vi "Main.vi"(8 "error in":errorcluster, 11 "Acquire in":refnum<class "DataAcquire Worker.lvclass">) -> (0 "error out":errorcluster, 3 "Acquire out":refnum<class "DataAcquire Worker.lvclass">)   [LabVIEW 2018, in "DataAcquire Worker.lvclass"]
doc: "The Queued Message Handler of a Worker."
uses:
  DataAcquire Worker.lvclass
  D:/Program Files (x86)/National Instruments/LabVIEW 2018/vi.lib/addons/_Workers/Library/Classes/Worker/Worker.lvclass
  DataAcquire Worker.lvclass/DataAcquire Worker.ctl
  Initialization Data.ctl
  <vilib>/addons/_Workers/Library/Classes/Message Queue/Message Queue.lvclass
  <vilib>/addons/_Workers/Library/Classes/Worker/Worker.lvclass/Worker.ctl
  DataSave Worker/DataSave Worker.lvclass
  <vilib>/addons/_Workers/Library/Classes/Message/Enqueue Message to Self v2.vi
  <vilib>/addons/_Workers/Library/Classes/Message/Enqueue Message to Queue.vi
  <vilib>/addons/_Workers/Library/Classes/Message/Message.lvclass
  ChartView Worker/ChartView Worker.lvclass
  D:/Program Files (x86)/National Instruments/LabVIEW 2018/vi.lib/addons/_Workers/Library/Classes/Workers Object/Workers Object.lvclass
  <vilib>/addons/_Workers/Library/Classes/Worker/Worker.lvclass
types:
  T1 = typedef "DataAcquire Worker.lvclass/Initialization Data.ctl" = cluster{"String":string, "Chart Queue":refnum<class "Message Queue.lvclass">}
  T2 = typedef "Workers.lvlib/Case Label.ctl" = string
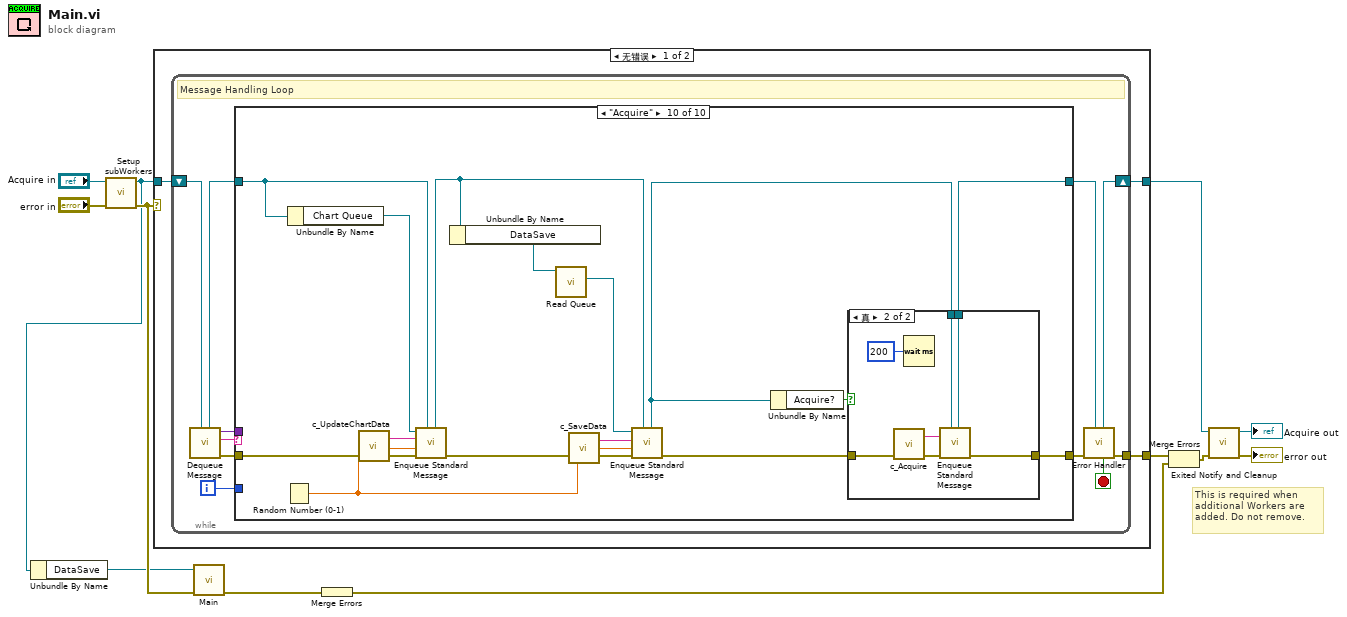
[diagram p0: block diagram]
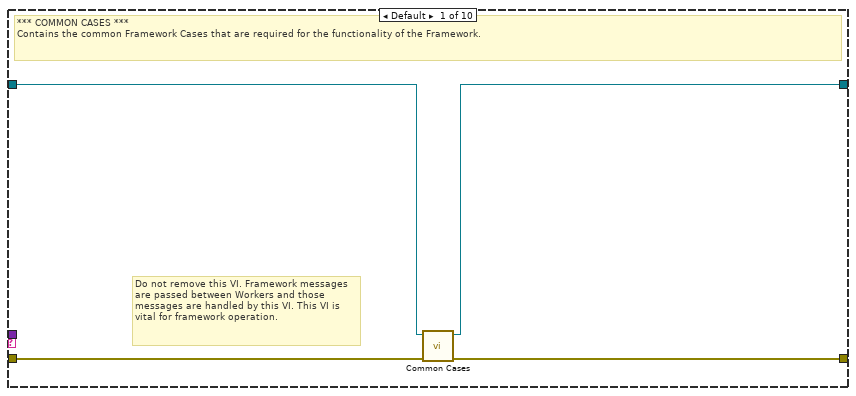
[diagram p2: hidden frame]
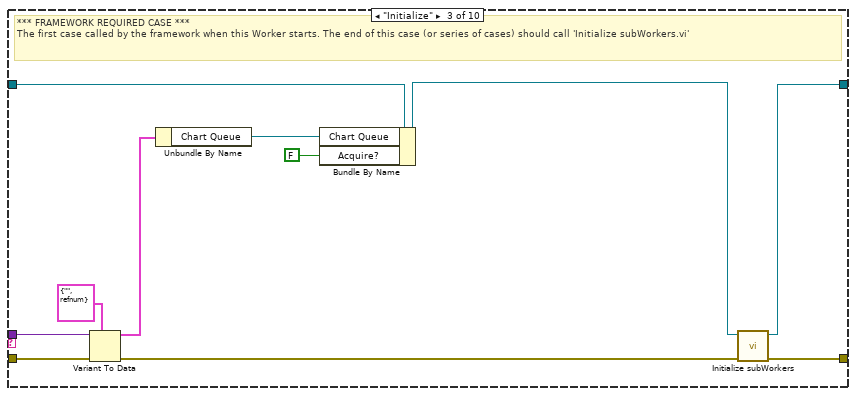
[diagram p4: hidden frame]
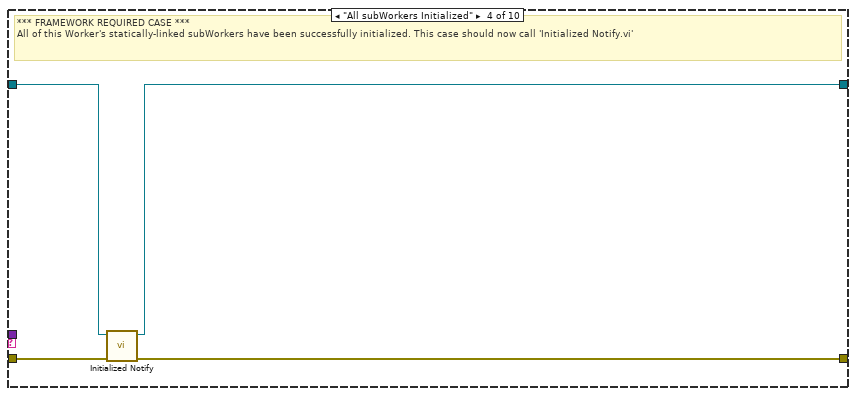
[diagram p5: hidden frame]
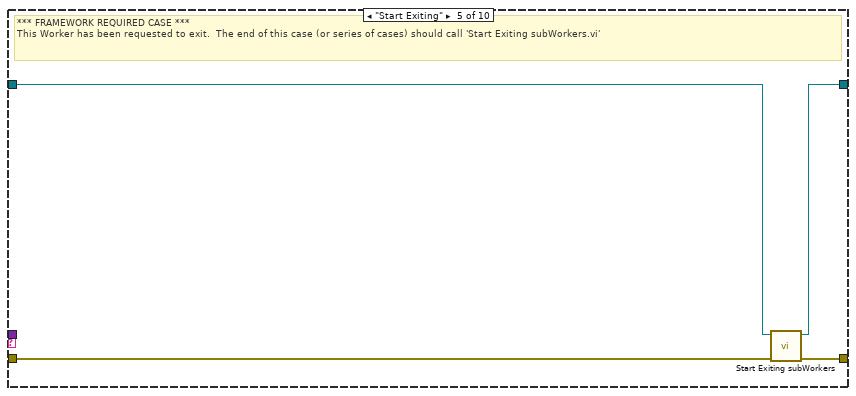
[diagram p6: hidden frame]
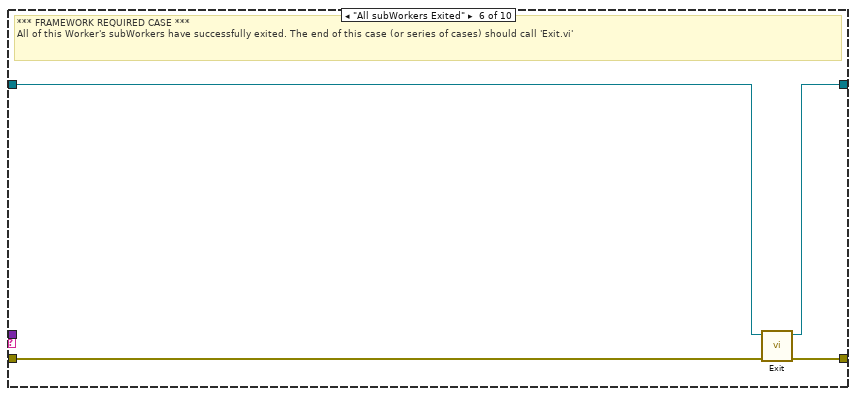
[diagram p7: hidden frame]
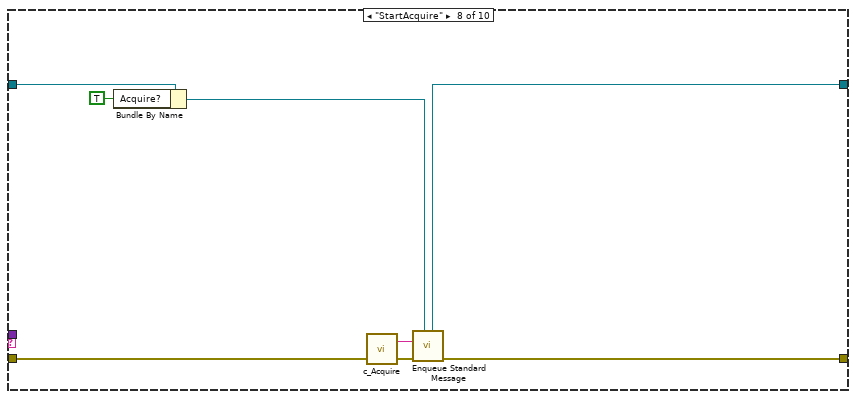
[diagram p9: hidden frame]
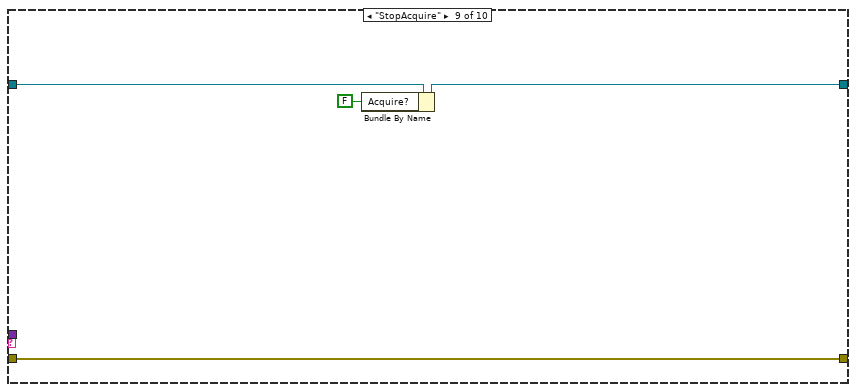
[diagram p10: hidden frame]
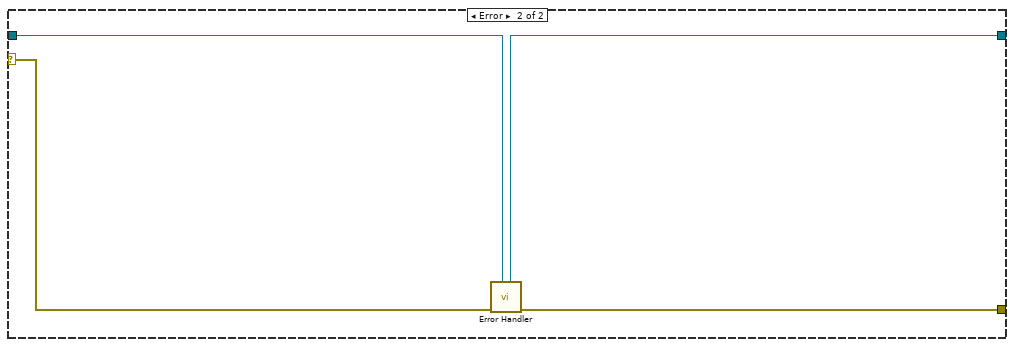
[diagram p12: hidden frame]
diagram:
  # "This is required when additional Workers are added. Do not remove."
  n1 = call "Setup subWorkers.vi"("error in"="error in", "DataAcquire Worker in"="Acquire in") -> ("error out"=w6:errorcluster, "DataAcquire Worker out"=w4:refnum<class "DataAcquire Worker.lvclass">)  [unwired: 8 in]
  n2 = Unbundle By Name(w4) -> ("DataSave"=w1:refnum<class "DataSave Worker.lvclass">)
  n3 = case shown="无错误" w6 {
    tunnel: w4 -> [w13 w93]
    tunnel: [w15 w94] -> w11
    tunnel: [w14 w92] -> w12
    selector: w6 -> [_ w95]
    frame No Error {
      n4 = while {
        shift-right: [w24] -> w14
        shift-left: w13 -> [w26]
        tunnel: [w25] -> w15
        i -> [w16]
        stop <- w17 stop-if-true
        # "Message Handling Loop"
        n5 = call-dynamic "Dequeue Message.vi"("Worker"=w26) -> ("error out"=w23:errorcluster, "Case out"=w18:string, "Data out"=w19:variant, "Worker out"=w21:refnum<class "DataAcquire Worker.lvclass">)  [unwired: 6 in, 1 out]
        n6 = case "Worker MHL Case Structure (DO NOT CHANGE LABEL NAME)" shown="\"Acquire\"" w18 {
          tunnel: w23 -> [w30 w31 w41 w47 w48 w55 w56 w64 w68 w78]
          tunnel: [w29 w31 w43 w45 w51 w54 w56 w61 w68 w83] -> w22
          tunnel: w21 -> [w28 w32 w40 w46 w49 w53 w57 w63 w67 w80]
          tunnel: [w27 w32 w42 w44 w50 w52 w57 w59 w66 w82] -> w20
          tunnel: w19 -> [_ _ w39 _ _ _ _ _ _ _]
          tunnel: w16 -> [_ _ _ _ _ _ _ _ _ _]
          frame Default {
            # "Do not remove this VI. Framework messages are passed between Workers and those messages are handled by this VI. This VI is vital for framework operation."
            # "*** COMMON CASES ***\nContains the common Framework Cases that are required for the functionality of the Framework."
            n7 = call-dynamic "Common Cases.vi"("error in"=w30, "Worker in"=w28) -> ("error out"=w29:errorcluster, "Worker out"=w27:refnum<class "DataAcquire Worker.lvclass">)  [unwired: 8 in]
          }
          frame "------ FRAMEWORK REQUIRED CASES ------" {
            # "Start of Framework Required Cases"
          }
          frame "Initialize" {
            # "*** FRAMEWORK REQUIRED CASE ***\nThe first case called by the framework when this Worker starts. The end of this case (or series of cases) should call 'Initialize subWorkers.vi'"
            n8 = Variant To Data(error in=w41, type=T1 {"String"="", "Chart Queue"=refnum} ("Cluster"), Variant=w39) -> (data=w36:T1, error out=w35:errorcluster)
            n9 = Unbundle By Name(w36) -> ("Chart Queue"=w34:refnum<class "Message Queue.lvclass">)
            n10 = Bundle By Name ("按名称捆绑")(cluster=w40, "Chart Queue"=w34, "Acquire?"=FALSE) -> (w37:refnum<class "DataAcquire Worker.lvclass">)
            n11 = call-dynamic "Initialize subWorkers.vi"("error in"=w35, "Worker"=w37) -> ("error out"=w43:errorcluster, "dup Worker out"=w42:refnum<class "DataAcquire Worker.lvclass">)  [unwired: 8 in]
          }
          frame "All subWorkers Initialized" {
            # "*** FRAMEWORK REQUIRED CASE ***\nAll of this Worker's statically-linked subWorkers have been successfully initialized. This case should now call 'Initialized Notify.vi'"
            n12 = call-dynamic "Initialized Notify.vi"("error in"=w47, "Worker"=w46) -> ("error out"=w45:errorcluster, "dup Worker out"=w44:refnum<class "DataAcquire Worker.lvclass">)  [unwired: 8 in]
          }
          frame "Start Exiting" {
            # "*** FRAMEWORK REQUIRED CASE ***\nThis Worker has been requested to exit.  The end of this case (or series of cases) should call 'Start Exiting subWorkers.vi'"
            n13 = call-dynamic "Start Exiting subWorkers.vi"("error_in"=w48, "Worker"=w49) -> ("error out"=w51:errorcluster, "dup Worker out"=w50:refnum<class "DataAcquire Worker.lvclass">)  [unwired: 8 in]
          }
          frame "All subWorkers Exited" {
            # "*** FRAMEWORK REQUIRED CASE ***\nAll of this Worker's subWorkers have successfully exited. The end of this case (or series of cases) should call 'Exit.vi'"
            n14 = call-dynamic "Exit.vi"("error_in"=w55, "Worker"=w53) -> ("error out"=w54:errorcluster, "dup Worker out"=w52:refnum<class "DataAcquire Worker.lvclass">)  [unwired: 8 in]
          }
          frame "-----------------------------------------------" {
            # "End of Framework Required Cases"
          }
          frame "StartAcquire" {
            n15 = Bundle By Name ("按名称捆绑")(cluster=w63, "Acquire?"=TRUE) -> (w60:refnum<class "DataAcquire Worker.lvclass">)
            n16 = call "c_Acquire.vi"() -> ("Case Label"=w58:T2)  [unwired: 1 in]
            n17 = call-poly <vilib>:"Enqueue Standard Message.vi"("Worker"=w60, "error in"=w64, "Case Label"=w58) -> ("error out"=w61:errorcluster, "dup Worker out"=w59:refnum<class "DataAcquire Worker.lvclass">)  [unwired: 7 in]
          }
          frame "StopAcquire" {
            n18 = Bundle By Name ("按名称捆绑")(cluster=w67, "Acquire?"=FALSE) -> (w66:refnum<class "DataAcquire Worker.lvclass">)
          }
          frame "Acquire" {
            n19 = Random Number (0-1)() -> (number: 0 to 1=w70:dbl)
            n20 = Unbundle By Name(w80) -> ("Chart Queue"=w79:refnum<class "Message Queue.lvclass">)
            n21 = call "c_UpdateChartData.vi"() -> ("Case Label"=w76:T2)  [unwired: 1 in]
            n22 = call-poly <vilib>:"Enqueue Standard Message.vi"("Worker"=w80, "error in"=w78, "Data"=w70, "Case Label"=w76, "Message Queue"=w79) -> ("error out"=w77:errorcluster, "dup Worker out"=w73:refnum<class "DataAcquire Worker.lvclass">)  [unwired: 4 in, 1 out]
            n23 = Unbundle By Name(w73) -> ("DataSave"=w72:refnum<class "DataSave Worker.lvclass">)
            n24 = call <vilib>:"Read Queue.vi"("Worker"=w72) -> ("Message Queue out"=w71:refnum<class "Message Queue.lvclass">)  [unwired: 9 in, 1 out]
            n25 = call "c_SaveData.vi"() -> ("Case Label"=w69:T2)  [unwired: 1 in]
            n26 = call-poly <vilib>:"Enqueue Standard Message.vi"("Worker"=w73, "error in"=w77, "Data"=w70, "Case Label"=w69, "Message Queue"=w71) -> ("error out"=w75:errorcluster, "dup Worker out"=w74:refnum<class "DataAcquire Worker.lvclass">)  [unwired: 4 in, 1 out]
            n27 = Unbundle By Name(w74) -> ("Acquire?"=w81:bool)
            n28 = case shown="真" w81 {
              tunnel: w74 -> [w84 w90]
              tunnel: w75 -> [w85 w89]
              tunnel: [w85 w88] -> w83
              tunnel: [w84 w87] -> w82
              frame False {
              }
              frame True {
                n29 = call "c_Acquire.vi"() -> ("Case Label"=w91:T2)  [unwired: 1 in]
                n30 = Wait (ms)(milliseconds to wait=u32 200 ("等待时间（毫秒）")) -> ()  [unwired: 1 out]
                n31 = call-poly <vilib>:"Enqueue Standard Message.vi"("Worker"=w90, "error in"=w89, "Case Label"=w91) -> ("error out"=w88:errorcluster, "dup Worker out"=w87:refnum<class "DataAcquire Worker.lvclass">)  [unwired: 7 in]
              }
            }
          }
        }
        n32 = call-dynamic "Error Handler.vi"("Worker"=w20, "error_in"=w22) -> ("error out"=w25:errorcluster, "Stop Loop"=w17:bool, "Worker out"=w24:refnum<class "DataAcquire Worker.lvclass">)  [unwired: 7 in]
      }
    }
    frame Error {
      n33 = call-dynamic "Error Handler.vi"("Worker"=w93, "error_in"=w95) -> ("error out"=w94:errorcluster, "Worker out"=w92:refnum<class "DataAcquire Worker.lvclass">)  [unwired: 7 in, 1 out]
    }
  }
  n34 = call-dynamic "Main.vi"("error in"=w6, "DataSave Worker in"=w1) -> ("error out"=w3:errorcluster)  [unwired: 8 in, 1 out]
  n35 = Merge Errors(w3) -> (w2:errorcluster)
  n36 = Merge Errors ("合并错误")(w11, w2) -> (w8:errorcluster)
  n37 = call-dynamic "Exited Notify and Cleanup.vi"("error_in"=w8, "Worker"=w12) -> ("error out"=→"error out":errorcluster, "dup Worker out"=→"Acquire out":refnum<class "DataAcquire Worker.lvclass">)  [unwired: 8 in]
